vi "Register gRPC Messages.vi"(8 "error in (no error)":errorcluster, 11 "gRPC ID":T1) -> (0 "error out":errorcluster, 3 "gRPC ID Out":T1)   [LabVIEW 2026, in "WebPageInterface_client.lvlib"]
uses:
  WebPageInterface_client.lvlib
  <vilib>/gRPC/LabVIEW gRPC Library/Shared/grpcId.ctl
  <vilib>/gRPC/LabVIEW gRPC Library/Server API/typeDefs/Message Metadata.ctl
  <vilib>/gRPC/LabVIEW gRPC Library/Server API/typeDefs/Message Element Metadata.ctl
  <vilib>/gRPC/LabVIEW gRPC Library/Server API/typeDefs/Message Element Type.ctl
  <vilib>/gRPC/LabVIEW gRPC Library/Server API/typeDefs/Enum Metadata.ctl
  <vilib>/gRPC/LabVIEW gRPC Library/grpc-lvsupport-release.lvlib
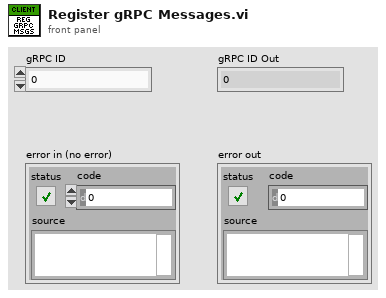
[diagram p1: front panel]
types:
  T1 = typedef "grpc-lvsupport-release.lvlib/grpcId.ctl" = u64
  T2 = typedef "grpc-lvsupport-release.lvlib/Enum Metadata.ctl" = cluster{"Version":i32, "Name":string, "Type Url":string, "Enum Values":string, "Allow Alias":bool}
  T3 = typedef "grpc-lvsupport-release.lvlib/Message Metadata.ctl" = cluster{"Version":i32, "Name":string, "Type Url":string, "Elements":T4[], "Has Oneof":bool}
  T4 = typedef "grpc-lvsupport-release.lvlib/Message Element Metadata.ctl" = cluster{"Field Name":string, "Embedded Message Name":string, "Protobuf Index":i32, "MessageElementType":T5, "Repeated":bool, "Is in Oneof":bool, "Oneof Container Name":string}
  T5 = typedef "grpc-lvsupport-release.lvlib/Message Element Type.ctl" = enum32{"Int32Value", "FloatValue", "DoubleValue", "BoolValue", "StringValue", "MessageValue", "Int64Value", "UInt32Value", "UInt64Value", "EnumValue", "Bytes", "Fixed64", "Fixed32", "SFixed64", "SFixed32", "SInt64", "SInt32"}
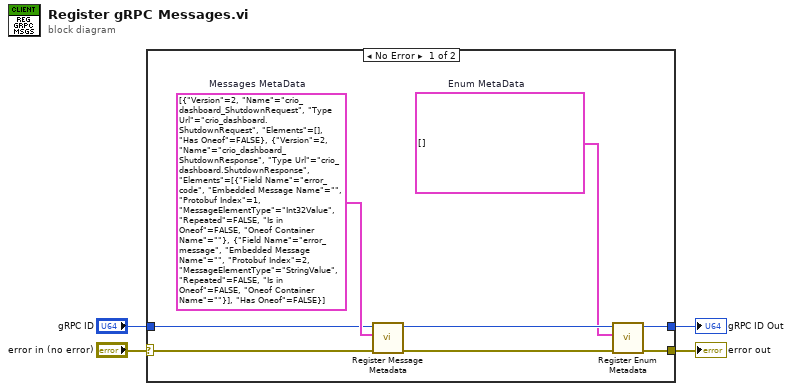
[diagram p0: block diagram]
diagram:
  n1 = case shown="No Error" "error in (no error)" {
    selector: "error in (no error)" -> [w10 w13]
    tunnel: [w9 w12] -> w1
    tunnel: [w6 w13] -> w4
    tunnel: "gRPC ID" -> [w9 w12]
    frame No Error {
      w5 = T2[] []  # Enum MetaData
      w11 = T3[] [{"Version"=2, "Name"="crio_dashboard_ShutdownRequest", "Type Url"="crio_dashboard.ShutdownRequest", "Elements"=[], "Has Oneof"=FALSE}, {"Version"=2, "Name"="crio_dashboard_ShutdownResponse", "Type Url"="crio_dashboard.ShutdownResponse", "Elements"=[{"Field Name"="error_code", "Embedded Message Name"="", "Protobuf Index"=1, "MessageElementType"=enum."Int32Value", "Repeated"=FALSE, "Is in Oneof"=FALSE, "Oneof Container Name"=""}, {"Field Name"="error_message", "Embedded Message Name"="", "Protobuf Index"=2, "MessageElementType"=enum."StringValue", "Repeated"=FALSE, "Is in Oneof"=FALSE, "Oneof Container Name"=""}], "Has Oneof"=FALSE}]  # Messages MetaData
      n2 = call <vilib>:"Register Message Metadata.vi"("error in"=w10, "Messages"=w11, "gRPCid in"=w9) -> ("error out"=w7:errorcluster, "gRPCid out"=w8:T1)  [unwired: 7 in]
      n3 = call <vilib>:"Register Enum Metadata.vi"("error in"=w7, "Enum Metadata"=w5, "gRPCid in"=w8) -> ("error out"=w6:errorcluster)  [unwired: 7 in, 1 out]
    }
    frame Error {
    }
  }
  "error out" <- w4
  "gRPC ID Out" <- w1
